vi "sub_main_log.vi"(8 "error in":errorcluster) -> (0 "error out":errorcluster)   [LabVIEW 2019]
uses:
  Ctrl/log_buffq.ctl
panel:
  out "i":i32
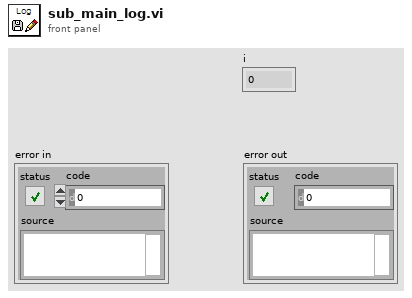
[diagram p1: front panel]
types:
  T1 = typedef "log_buffq.ctl" = enum16{"create", "write", "read", "close"}
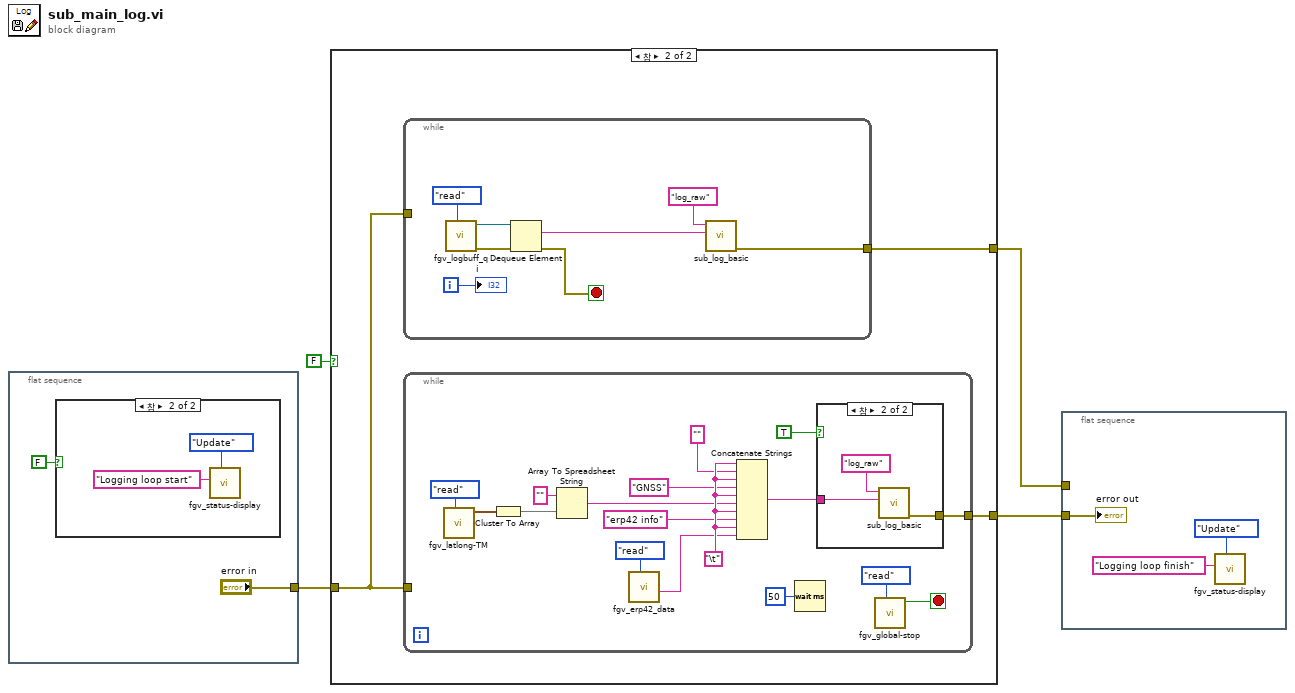
[diagram p0: block diagram]
diagram:
  n1 = flat-sequence {
    tunnel: ["error in"] -> w3
    frame #0 {
      n2 = case shown="참" FALSE {
        frame False {
        }
        frame True {
          n3 = call "fgv_status-display.vi"("Mode"=enum16{"Initial", "Update", "Clear"}."Update", "title"="Logging loop start" ("String in 1")) -> ()  [unwired: 9 in, 1 out]
        }
      }
    }
  }
  n4 = case shown="참" FALSE {
    tunnel: [_ w11] -> w4
    tunnel: w3 -> [_ w10]
    tunnel: [_ w9] -> w2
    frame False {
    }
    frame True {
      n5 = while {
        tunnel: w10 -> [_]
        tunnel: [w12] -> w9
        i -> [w15]
        stop <- w16 stop-if-true
        n6 = call "fgv_logbuff_q.vi"("cmd"=log_buffq."read") -> ("error out"=w17:errorcluster, "queue out"=w18:refnum<queue>)  [unwired: 9 in]
        n7 = Dequeue Element(queue=w18, error in (no error)=w17) -> (element=w13:string, error out=w16:errorcluster)  [unwired: 1 in, 2 out]
        n8 = call "sub_log_basic.vi"("desc"=w13, "Title"="log_raw") -> ("error out"=w12:errorcluster)  [unwired: 9 in]
        "i" <- w15
      }
      n9 = while {
        tunnel: w10 -> [_]
        tunnel: [w31] -> w11
        stop <- w28 stop-if-true
        w35 = "\t"
        n10 = call "fgv_latlong-TM.vi"("cmd"=enum16{"write", "read"}."read") -> ("latlong out"=w20:cluster{"lat":dbl, "long":dbl})  [unwired: 9 in, 1 out]
        n11 = Cluster To Array(cluster=w20) -> (array=w23:dbl[])
        n12 = Array To Spreadsheet String(array=w23, 3:"" ("포맷 문자열")) -> (spreadsheet string=w21:string)  [unwired: 1 in]
        n13 = call "fgv_erp42_data.vi"("cmd"=enum16{"init", "read", "write"}."read") -> ("erp recv out"=w25:string)  [unwired: 8 in, 2 out]
        n14 = Concatenate Strings(w35, "" ("포맷 문자열"), w35, "GNSS" ("포맷 문자열"), w35, w21, w35, "erp42 info" ("문자열"), w35, w25) -> (w36:string)
        n15 = Wait (ms)(milliseconds to wait=u32 50) -> ()  [unwired: 1 out]
        n16 = case shown="참" TRUE {
          tunnel: w36 -> [_ w39]
          tunnel: [_ w37] -> w31
          frame False {
          }
          frame True {
            n17 = call "sub_log_basic.vi"("desc"=w39, "Title"="log_raw") -> ("error out"=w37:errorcluster)  [unwired: 9 in]
          }
        }
        n18 = call "fgv_global-stop.vi"("cmd"=enum16{"init", "stop", "read"}."read") -> ("val_out"=w28:bool)  [unwired: 10 in]
      }
    }
  }
  n19 = flat-sequence {
    tunnel: w4 -> [w42]
    tunnel: w2 -> [_]
    frame #0 {
      n20 = call "fgv_status-display.vi"("Mode"=enum16{"Initial", "Update", "Clear"}."Update", "title"="Logging loop finish" ("String in 1")) -> ()  [unwired: 9 in, 1 out]
      "error out" <- w42
    }
  }
